vi "PointToWheelAngle.vi"(6 "Wheel Number":dbl, 7 "JoystickIn":i32[](array[slide]) scale=-37626.0..37626.0, 8 "Yw":dbl, 9 "Xw":dbl, 10 "y":dbl, 11 "x":dbl) -> (2 "Radius":dbl, 3 "Desired Angle":dbl)   [LabVIEW 2013, in "ProcessorHelperFunctions.lvlib"]
uses:
  ProcessorHelperFunctions.lvlib
  <vilib>/Analysis/coordinate.llb/Angle Range (Degree).ctl
  <vilib>/Analysis/coordinate.llb/Angle Units.ctl
  <vilib>/Analysis/coordinate.llb/Wrap Angle (scalar).vi
  <vilib>/Analysis/NI_AAL_Angle.lvlib
panel:
  # "(x, y) is the desired\npivot point in space\nwith respect to the \nrobot."
  # "Xw is x distance between the\nwheels on the robot"
  # "Yw is y distance between the\nwheels on the robot"
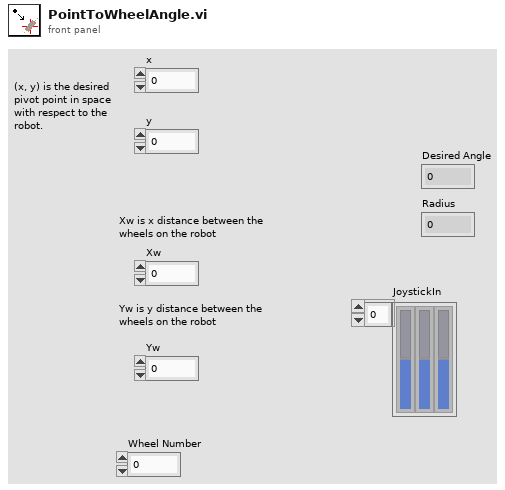
[diagram p1: front panel]
types:
  T1 = cluster{"JoystickIn[0]":i32, "JoystickIn[1]":i32, "JoystickIn[2]":i32, "JoystickIn[3]":i32, "JoystickIn[4]":i32, "JoystickIn[5]":i32, "JoystickIn[6]":i32, "JoystickIn[7]":i32, "JoystickIn[8]":i32}
  T2 = typedef "NI_AAL_Angle.lvlib/Angle Units.ctl" = i32
  T3 = typedef "NI_AAL_Angle.lvlib/Angle Range (Degree).ctl" = u16
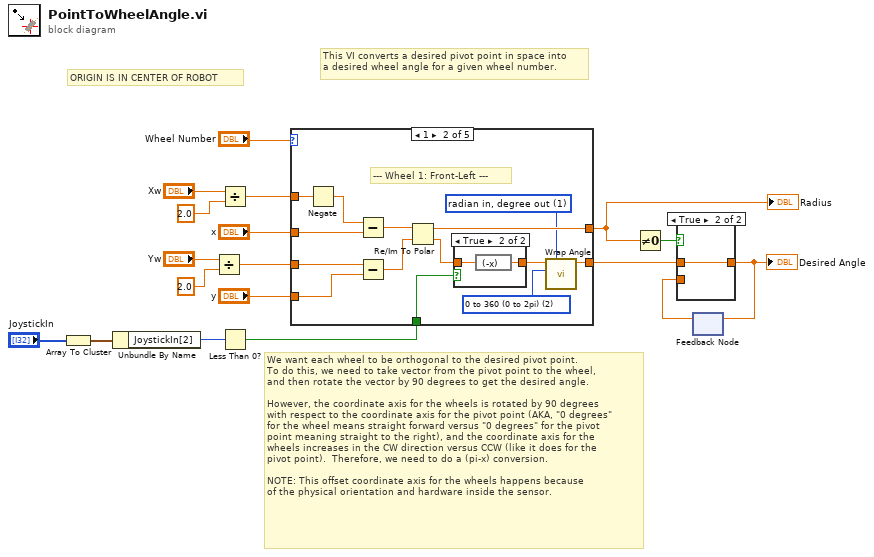
[diagram p0: block diagram]
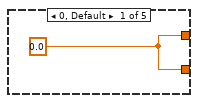
[diagram p3: hidden frame]
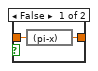
[diagram p4: hidden frame]
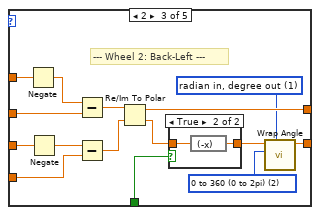
[diagram p5: hidden frame]
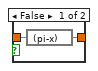
[diagram p6: hidden frame]
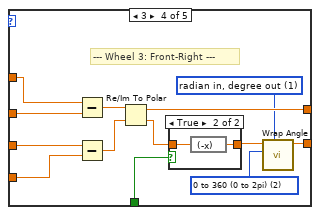
[diagram p7: hidden frame]
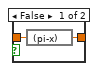
[diagram p8: hidden frame]
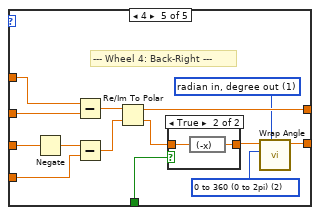
[diagram p9: hidden frame]
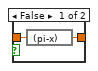
[diagram p10: hidden frame]
diagram:
  # "We want each wheel to be orthogonal to the desired pivot point.\nTo do this, we need to take vector from the pivot point to the wheel, \nand then rotate the vector by 90 degrees to get the desired angle.  \n\nHowever, the coordinate axis for the wheels is rotated by 90 degrees \nwith respect to the coordinate axis for the pivot point (AKA, \"0 degrees\"\nfor the wheel means straight forward versus \"0 degrees\" for the pivot\npoint meaning straight to the right), and the coordinate axis for the \nwheels increases in the CW direction versus CCW (like it does for the \npivot point).  Therefore, we need to do a (pi-x) conversion.\n\nNOTE: This offset coordinate axis for the wheels happens because\nof the physical orientation and hardware inside the sensor."
  # "This VI converts a desired pivot point in space into\na desired wheel angle for a given wheel number."
  # "ORIGIN IS IN CENTER OF ROBOT"
  n1 = Array To Cluster(array="JoystickIn") -> (cluster=w4:T1)
  n2 = Unbundle By Name(w4) -> ("JoystickIn[2]"=w2:i32)
  n3 = Divide(x="Yw", y=2.0) -> (x/y=w6:dbl)
  n4 = Divide(x="Xw", y=2.0) -> (x/y=w8:dbl)
  n5 = Less Than 0?(x=w2) -> (x < 0?=w1:bool)
  n6 = case shown="1" "Wheel Number" {
    tunnel: w8 -> [_ w30 w48 w64 w81]
    tunnel: "x" -> [_ w29 w47 w67 w85]
    tunnel: "y" -> [_ w28 w45 w66 w84]
    tunnel: w6 -> [_ w27 w46 w65 w83]
    tunnel: [w19 w25 w43 w62 w79] -> w11
    tunnel: [w19 w26 w44 w63 w80] -> w13
    tunnel: w1 -> [_ w20 w38 w57 w74]
    frame 0, Default {
      w19 = 0.0 ("rotated angle")
    }
    frame 1 {
      w23 = T2 1 items=["radian in, radian out", "radian in, degree out", "degree in, degree out", "degree in, radian out"] ("angle units")
      w24 = T3 2 items=["none", "-180 to 180 (-pi to pi)", "0 to 360 (0 to 2pi)"] ("rotated angle range")
      # "--- Wheel 1: Front-Left ---"
      n7 = Negate(x=w30) -> (-x=w31:dbl)
      n8 = Subtract(x=w31, y=w29) -> (x-y=w33:dbl)
      n9 = Subtract(x=w27, y=w28) -> (x-y=w32:dbl)
      n10 = Re/Im To Polar(2:w32, 3:w33) -> (0:w22:dbl, 1:w26:dbl)
      n11 = case shown="True" w20 {
        tunnel: w22 -> [w35 w36]
        tunnel: [w34 w37] -> w21
        frame False {
          n12 = expression code="(pi-x)"(w35) -> (w34:dbl)
        }
        frame True {
          n13 = expression code="(-x)"(w36) -> (w37:dbl)
        }
      }
      n14 = call-poly <vilib>:"Wrap Angle.vi"("angle units"=w23, "angle range"=w24, "angle in"=w21) -> ("angle out"=w25:dbl)  [unwired: 7 in, 1 out]
    }
    frame 2 {
      w42 = T2 1 items=["radian in, radian out", "radian in, degree out", "degree in, degree out", "degree in, radian out"] ("angle units")
      w41 = T3 2 items=["none", "-180 to 180 (-pi to pi)", "0 to 360 (0 to 2pi)"] ("rotated angle range")
      # "--- Wheel 2: Back-Left ---"
      n15 = Negate(x=w48) -> (-x=w50:dbl)
      n16 = Negate(x=w46) -> (-x=w49:dbl)
      n17 = Subtract(x=w50, y=w47) -> (x-y=w52:dbl)
      n18 = Subtract(x=w49, y=w45) -> (x-y=w51:dbl)
      n19 = Re/Im To Polar(2:w51, 3:w52) -> (0:w39:dbl, 1:w44:dbl)
      n20 = case shown="True" w38 {
        tunnel: w39 -> [w54 w55]
        tunnel: [w53 w56] -> w40
        frame False {
          n21 = expression code="(pi-x)"(w54) -> (w53:dbl)
        }
        frame True {
          n22 = expression code="(-x)"(w55) -> (w56:dbl)
        }
      }
      n23 = call-poly <vilib>:"Wrap Angle.vi"("angle units"=w42, "angle range"=w41, "angle in"=w40) -> ("angle out"=w43:dbl)  [unwired: 7 in, 1 out]
    }
    frame 3 {
      w60 = T2 1 items=["radian in, radian out", "radian in, degree out", "degree in, degree out", "degree in, radian out"] ("angle units")
      w61 = T3 2 items=["none", "-180 to 180 (-pi to pi)", "0 to 360 (0 to 2pi)"] ("rotated angle range")
      # "--- Wheel 3: Front-Right ---"
      n24 = Subtract(x=w64, y=w67) -> (x-y=w68:dbl)
      n25 = Subtract(x=w65, y=w66) -> (x-y=w69:dbl)
      n26 = Re/Im To Polar(2:w69, 3:w68) -> (0:w58:dbl, 1:w63:dbl)
      n27 = case shown="True" w57 {
        tunnel: w58 -> [w71 w72]
        tunnel: [w70 w73] -> w59
        frame False {
          n28 = expression code="(pi-x)"(w71) -> (w70:dbl)
        }
        frame True {
          n29 = expression code="(-x)"(w72) -> (w73:dbl)
        }
      }
      n30 = call-poly <vilib>:"Wrap Angle.vi"("angle units"=w60, "angle range"=w61, "angle in"=w59) -> ("angle out"=w62:dbl)  [unwired: 7 in, 1 out]
    }
    frame 4 {
      w77 = T2 1 items=["radian in, radian out", "radian in, degree out", "degree in, degree out", "degree in, radian out"] ("angle units")
      w78 = T3 2 items=["none", "-180 to 180 (-pi to pi)", "0 to 360 (0 to 2pi)"] ("rotated angle range")
      # "--- Wheel 4: Back-Right ---"
      n31 = Negate(x=w83) -> (-x=w82:dbl)
      n32 = Subtract(x=w81, y=w85) -> (x-y=w86:dbl)
      n33 = Subtract(x=w82, y=w84) -> (x-y=w87:dbl)
      n34 = Re/Im To Polar(2:w87, 3:w86) -> (0:w75:dbl, 1:w80:dbl)
      n35 = case shown="True" w74 {
        tunnel: w75 -> [w89 w90]
        tunnel: [w88 w91] -> w76
        frame False {
          n36 = expression code="(pi-x)"(w89) -> (w88:dbl)
        }
        frame True {
          n37 = expression code="(-x)"(w90) -> (w91:dbl)
        }
      }
      n38 = call-poly <vilib>:"Wrap Angle.vi"("angle units"=w77, "angle range"=w78, "angle in"=w76) -> ("angle out"=w79:dbl)  [unwired: 7 in, 1 out]
    }
  }
  "Radius" <- w13
  n39 = Not Equal To 0?(x=w13) -> (x != 0?=w12:bool)
  n40 = feedback #1() -> (w10:dbl)  [unwired: 1 in]
  n41 = case shown="True" w12 {
    tunnel: w11 -> [_ w93]
    tunnel: w10 -> [w92 _]
    tunnel: [w92 w93] -> w9
    frame False {
    }
    frame True {
    }
  }
  "Desired Angle" <- w9
  n42 = feedback-in #1(w9) -> ()
